vi "Eulogy.vi"(6 "Mouse Position":T1, 7 "User VI Ref":refnum<vi>, 8 "Is Multi-select?":bool, 9 "Remaining Items":refnum<vi>[](array[refnum]), 10 "Affected Items":T8, 11 "Menu Refnum":refnum<k9>) -> (3 "Menu Items To Add":T2[](array[typedef]))   [LabVIEW 2017, in "Shortcut Menu.lvlib"]
doc: "This VI is part of a plug-in for modifying the LabVIEW shortcut menus. This is the builder VI which is called when the shortcut menu is built. It tells LabVIEW which shortcut menu items to add to the menu."
uses:
  Shortcut Menu.lvlib
  <resource>/plugins/PopupMenus/support/Shortcut Menu Item Definition.ctl
  <resource>/plugins/PopupMenus/support/Transaction Control.ctl
  <resource>/plugins/PopupMenus/support/Position In Menu.ctl
  <resource>/plugins/PopupMenus/support/Relative Position.ctl
  <resource>/plugins/PopupMenus/support/Checkmark Status.ctl
  <resource>/plugins/PopupMenus/support/Enabled Menu Item Status.ctl
  Eulogy.ctl
  <vilib>/Utility/miscctls.llb/LVPositionTypeDef.ctl
  Toolkit VIs/Toolkit VIs.lvlib
panel:
  # "Rules a popup plug-in must follow:\n* This VI's file name must match the file name of the LLB -- only the file extensions should be different.\n* This VI must have debugging disabled or it will be ignored as a plug-in.\n* For all menu items, \"tag suffix + file name of this VI\" must be less than 240 characters.\n* You can disconnect the \"Affected Items\" from the typedef to make the plug-in load faster. The typedef is only there to assist you in keeping this VI and the execution VI using to the same type.\n* All controls on this panel except \"Affected Items\" are locked to prevent accidental edits. Do not change the types or the names of controls other than the elements inside the \"Affected Items\" cluster.\n* See Context Help for more information on the individual controls."
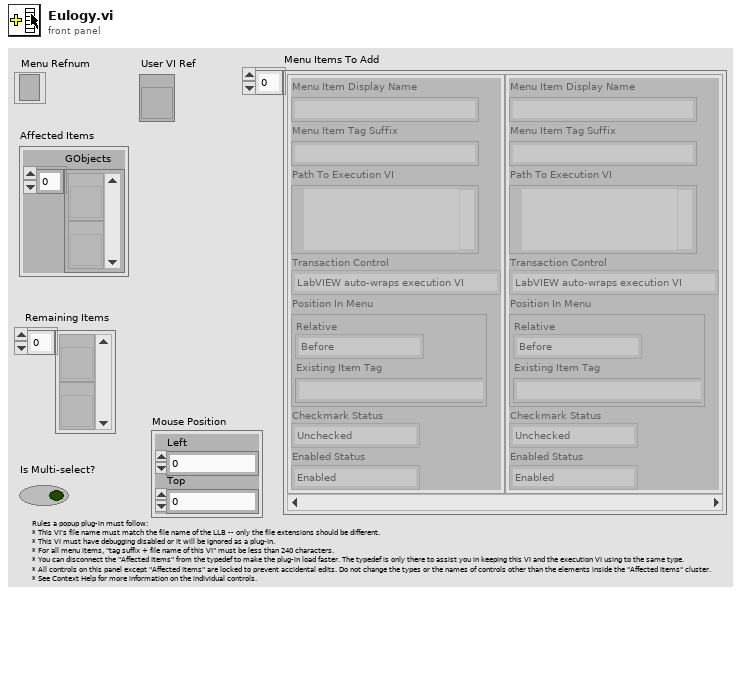
[diagram p1: front panel]
types:
  T1 = typedef "LVPositionTypeDef.ctl" = cluster{"Left":i32, "Top":i32}
  T2 = typedef "Shortcut Menu Item Definition.ctl" = cluster{"Menu Item Display Name":string, "Menu Item Tag Suffix":string, "Path To Execution VI":path, "Transaction Control":T3, "Position In Menu":T4, "Checkmark Status":T6, "Enabled Status":T7}
  T3 = typedef "Transaction Control.ctl" = enum8{"LabVIEW auto-wraps execution VI", "Execution VI will define if needed"}
  T4 = typedef "Position In Menu.ctl" = cluster{"Relative":T5, "Existing Item Tag":string}
  T5 = typedef "Relative Position.ctl" = enum8{"Before", "Instead of", "After", "Into Submenu"}
  T6 = typedef "Checkmark Status.ctl" = enum8{"Unchecked", "Checked"}
  T7 = typedef "Enabled Menu Item Status.ctl" = enum8{"Enabled", "Disabled"}
  T8 = typedef "Shortcut Menu.lvlib/Eulogy.ctl" = cluster{"GObjects":refnum<vi>[]}
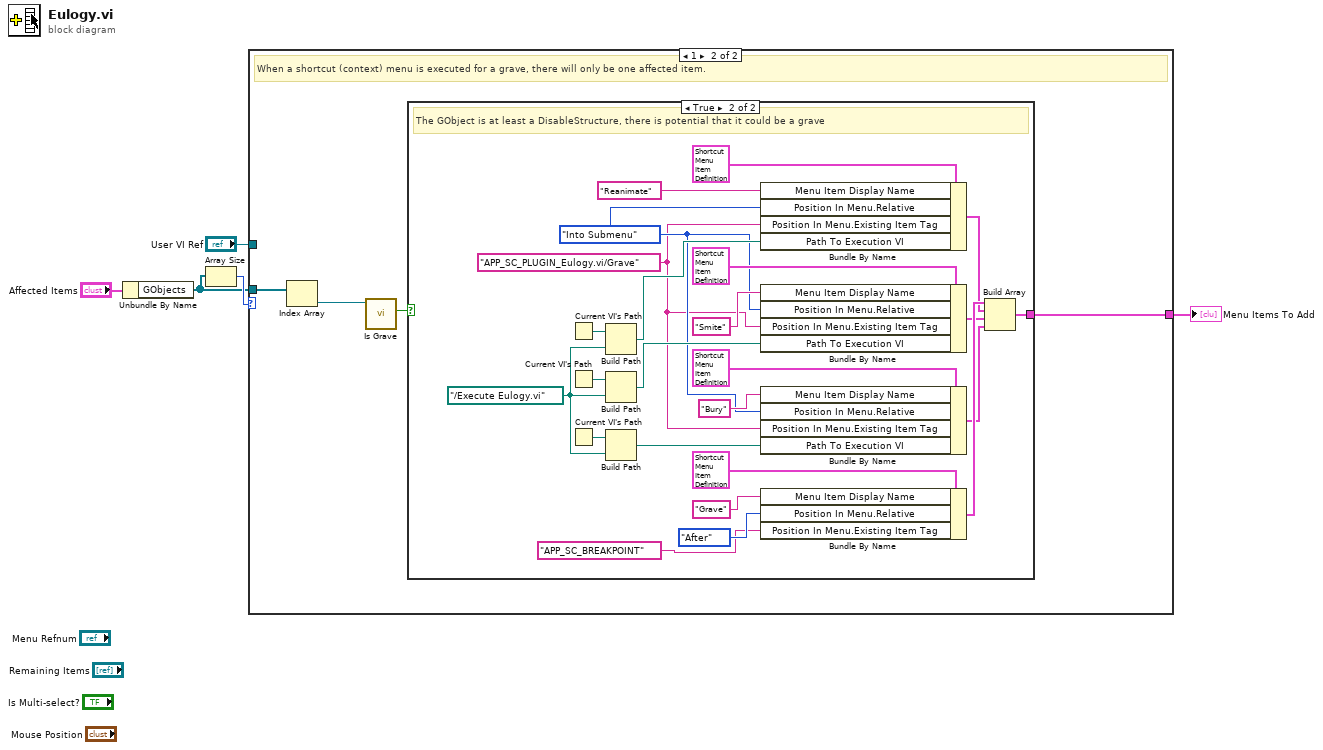
[diagram p0: block diagram]
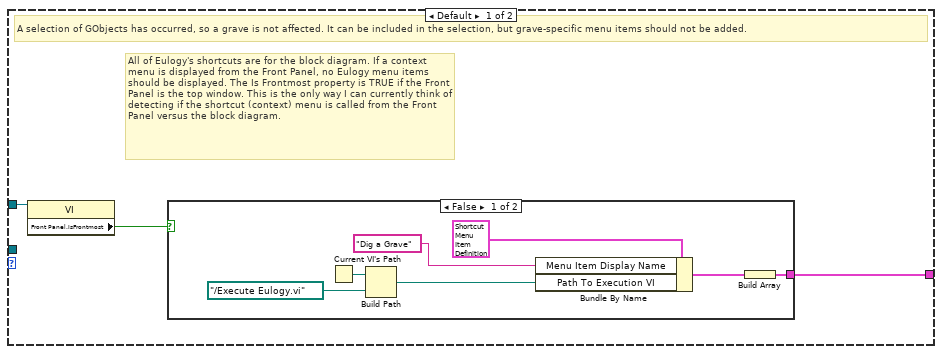
[diagram p2: hidden frame]
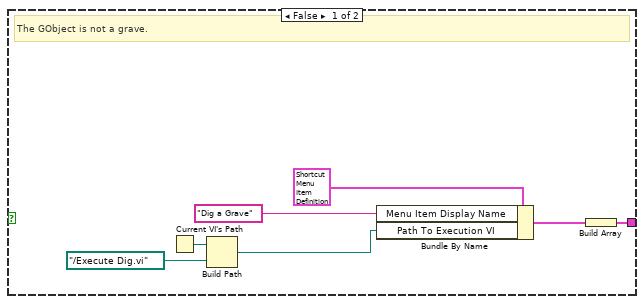
[diagram p4: hidden frame]
diagram:
  n1 = Unbundle By Name("Affected Items") -> ("GObjects"=w3:refnum<vi>[])
  n2 = Array Size(array=w3) -> (size(s)=w4:i32)
  n3 = case shown="1" w4 {
    tunnel: w3 -> [_ w19]
    tunnel: [w8 w18] -> w2
    tunnel: "User VI Ref" -> [w7 _]
    frame Default {
      # "All of Eulogy's shortcuts are for the block diagram. If a context menu is displayed from the Front Panel, no Eulogy menu items should be displayed. The Is Frontmost property is TRUE if the Front Panel is the top window. This is the only way I can currently think of detecting if the shortcut (context) menu is called from the Front Panel versus the block diagram."
      # "A selection of GObjects has occurred, so a grave is not affected. It can be included in the selection, but grave-specific menu items should not be added."
      n4 = property class="VI"(reference=w7) -> ("Front Panel.IsFrontmost"=w6:bool)  [unwired: 1 in, 2 out]
      n5 = case shown="False" w6 {
        tunnel: [w9 _] -> w8
        frame False {
          n6 = Current VI's Path() -> (path=w12:path)
          n7 = Build Path(base path=w12, name or relative path=path "../Execute Eulogy.vi" ("execute path")) -> (appended path=w11:path)
          n8 = Bundle By Name(cluster=T2 {"Menu Item Display Name"="", "Menu Item Tag Suffix"="", "Path To Execution VI"=path "", "Transaction Control"=enum."LabVIEW auto-wraps execution VI", "Position In Menu"={"Relative"=enum."Before", "Existing Item Tag"=""}, "Checkmark Status"=enum."Unchecked", "Enabled Status"=enum."Enabled"} ("Cluster"), "Menu Item Display Name"="Dig a Grave", "Path To Execution VI"=w11) -> (w10:T2)
          n9 = Build Array(w10) -> (w9:T2[])
        }
        frame True {
        }
      }
    }
    frame 1 {
      # "When a shortcut (context) menu is executed for a grave, there will only be one affected item."
      n10 = Index Array(array=w19) -> (element=w17:refnum<vi>)  [unwired: 1 in]
      n11 = call "Is Grave.vi"("GObject In"=w17) -> ("Grave?"=w16:bool)  [unwired: 8 in, 2 out]
      n12 = case shown="True" w16 {
        tunnel: [w26 w50] -> w18
        frame False {
          # "The GObject is not a grave."
          n13 = Current VI's Path() -> (path=w22:path)
          n14 = Build Path(base path=w22, name or relative path=path "../Execute Dig.vi" ("execute path")) -> (appended path=w21:path)
          n15 = Bundle By Name(cluster=T2 {"Menu Item Display Name"="", "Menu Item Tag Suffix"="", "Path To Execution VI"=path "", "Transaction Control"=enum."LabVIEW auto-wraps execution VI", "Position In Menu"={"Relative"=enum."Before", "Existing Item Tag"=""}, "Checkmark Status"=enum."Unchecked", "Enabled Status"=enum."Enabled"} ("Cluster"), "Menu Item Display Name"="Dig a Grave", "Path To Execution VI"=w21) -> (w20:T2)
          n16 = Build Array(w20) -> (w26:T2[])
        }
        frame True {
          w33 = "APP_SC_PLUGIN_Eulogy.vi/Grave" ("Position In Menu.Existing Item Tag")
          w27 = path "../Execute Eulogy.vi" ("execute path")
          w34 = Relative_Position."Into Submenu" ("Position In Menu.Relative")
          # "The GObject is at least a DisableStructure, there is potential that it could be a grave"
          n17 = Current VI's Path() -> (path=w41:path)
          n18 = Current VI's Path() -> (path=w37:path)
          n19 = Current VI's Path() -> (path=w45:path)
          n20 = Build Path(base path=w41, name or relative path=w27) -> (appended path=w40:path)
          n21 = Build Path(base path=w37, name or relative path=w27) -> (appended path=w36:path)
          n22 = Build Path(base path=w45, name or relative path=w27) -> (appended path=w44:path)
          n23 = Bundle By Name(cluster=T2 {"Menu Item Display Name"="", "Menu Item Tag Suffix"="", "Path To Execution VI"=path "", "Transaction Control"=enum."LabVIEW auto-wraps execution VI", "Position In Menu"={"Relative"=enum."Before", "Existing Item Tag"=""}, "Checkmark Status"=enum."Unchecked", "Enabled Status"=enum."Enabled"} ("Cluster"), "Menu Item Display Name"="Reanimate", "Position In Menu.Relative"=w34, "Position In Menu.Existing Item Tag"=w33, "Path To Execution VI"=w40) -> (w30:T2)
          n24 = Bundle By Name(cluster=T2 {"Menu Item Display Name"="", "Menu Item Tag Suffix"="", "Path To Execution VI"=path "", "Transaction Control"=enum."LabVIEW auto-wraps execution VI", "Position In Menu"={"Relative"=enum."Before", "Existing Item Tag"=""}, "Checkmark Status"=enum."Unchecked", "Enabled Status"=enum."Enabled"} ("Cluster"), "Menu Item Display Name"="Smite", "Position In Menu.Relative"=w34, "Position In Menu.Existing Item Tag"=w33, "Path To Execution VI"=w36) -> (w29:T2)
          n25 = Bundle By Name(cluster=T2 {"Menu Item Display Name"="", "Menu Item Tag Suffix"="", "Path To Execution VI"=path "", "Transaction Control"=enum."LabVIEW auto-wraps execution VI", "Position In Menu"={"Relative"=enum."Before", "Existing Item Tag"=""}, "Checkmark Status"=enum."Unchecked", "Enabled Status"=enum."Enabled"} ("Cluster"), "Menu Item Display Name"="Bury", "Position In Menu.Relative"=w34, "Position In Menu.Existing Item Tag"=w33, "Path To Execution VI"=w44) -> (w28:T2)
          n26 = Bundle By Name(cluster=T2 {"Menu Item Display Name"="", "Menu Item Tag Suffix"="", "Path To Execution VI"=path "", "Transaction Control"=enum."LabVIEW auto-wraps execution VI", "Position In Menu"={"Relative"=enum."Before", "Existing Item Tag"=""}, "Checkmark Status"=enum."Unchecked", "Enabled Status"=enum."Enabled"} ("Cluster"), "Menu Item Display Name"="Grave", "Position In Menu.Relative"=Relative_Position."After", "Position In Menu.Existing Item Tag"="APP_SC_BREAKPOINT") -> (w35:T2)
          n27 = Build Array(w35, w30, w29, w28) -> (w50:T2[])
        }
      }
    }
  }
  "Menu Items To Add" <- w2
